vi "Error Injector.vi"(10 "Error?":bool, 11 "Semiconductor Module Context":T1) -> (0 "error out":errorcluster, 3 "Output":dbl)   [LabVIEW 2018]
uses:
  <vilib>/NI_TestStand_SemiconductorModule/NI_TestStand_Semiconductor_Module.lvlibp/PinMap/General/SemiconductorModuleContext.ctl
  <vilib>/Utility/error.llb/Error Cluster From Error Code.vi
  <vilib>/ErrorRing/Error Ring.xnode
  <vilib>/NI_TestStand_SemiconductorModule/NI_TestStand_Semiconductor_Module.lvlibp
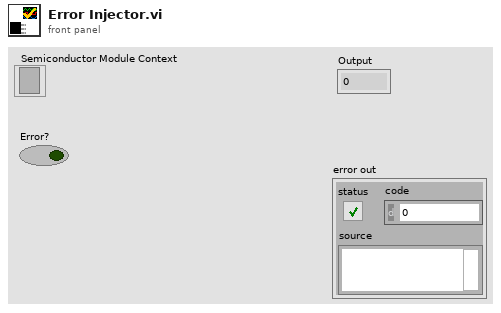
[diagram p1: front panel]
types:
  T1 = typedef "NI_TestStand_Semiconductor_Module.lvlibp/SemiconductorModuleContext.ctl" = refnum<k7>
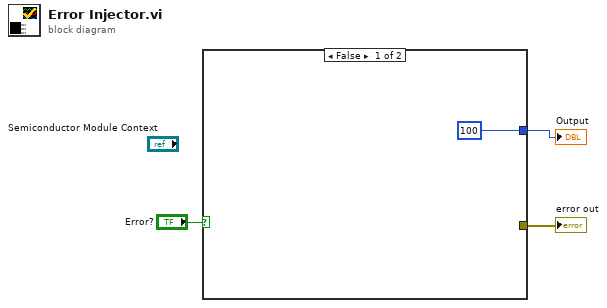
[diagram p0: block diagram]
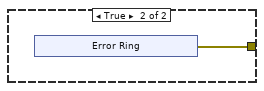
[diagram p2: hidden frame]
diagram:
  n1 = case shown="False" "Error?" {
    tunnel: [_ w5] -> w2
    tunnel: [100 _] -> w1
    frame False {
    }
    frame True {
      n2 = xnode "Error Ring"() -> ("error out"=w5:errorcluster)
    }
  }
  "error out" <- w2
  "Output" <- w1
